vi "Pre Launch Init.vi"(11 "CS++DeviceGUIActor in":refnum<class "CS++DeviceGUIActor.lvclass">) -> (0 "error out":errorcluster, 3 "CS++DeviceGUIActor out":refnum<class "CS++DeviceGUIActor.lvclass">)   [LabVIEW 2013, in "CS++DeviceGUIActor.lvlib" / "CS++DeviceGUIActor.lvclass"]
doc: "(<B>Filename</B>: Actor Framework.lvlib:Actor.lvclass:Pre Launch Init.vi)\n\nDefines behavior that occurs after the Launch Actor method is invoked but before the actor's Actor Core method begins running.\n\nThe Pre Launch Init method is guaranteed to finish before the Launch Actor method returns to its caller and before the actor itself receives any messages. Any references that the Pre Launch Init method obtains are guaranteed to have the same lifetime as the actor itself. Any errors that the Pre Launch Init method returns will abort the launch.\n\nBy default, this method does nothing. A descendant class may override it to define behavior."
uses:
  CS++DeviceGUIActor.lvclass
  CS++GUIActor/CS++GUIActor.lvclass
  CS++BaseActor/CS++BaseActor.lvclass/CS++BaseActor.ctl
  Classes/CS++BaseClasses/Factory/CS++Factory.lvclass
  Classes/CS++ProcessVariables/PVConnection/PVConnection.lvclass
  Classes/CS++ProcessVariables/SVConnection/SVConnection.lvclass
  Classes/CS++ProcessVariables/PVConnection/PVConnection.lvclass/PVConnection.ctl
  Classes/CS++ProcessVariables/ProcessVariable/PV.lvclass/PV.ctl
  CS++DeviceGUIActor.lvclass/CS++DeviceGUIActor.ctl
  Classes/CS++ProcessVariables/ProcessVariable/Read Data.vi
  CS++BaseActor/Read CS++Factory.vi
  Classes/CS++ProcessVariables/ProcessVariable/PV.lvclass
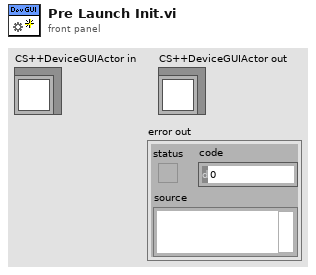
[diagram p1: front panel]
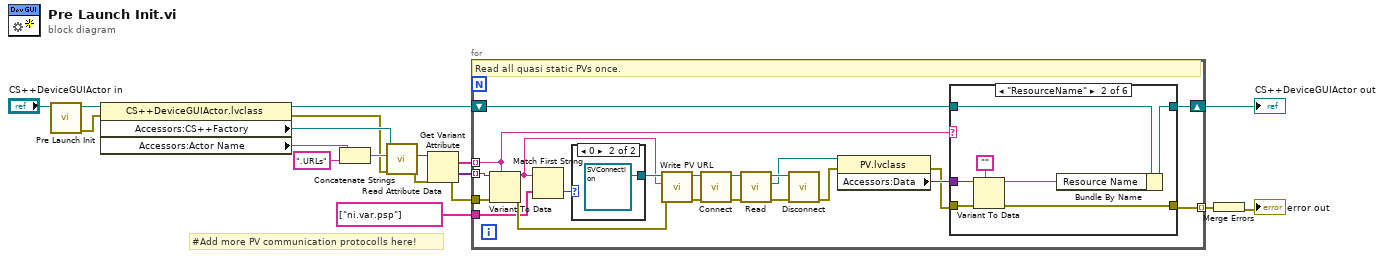
[diagram p0: block diagram]
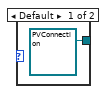
[diagram p2: hidden frame]
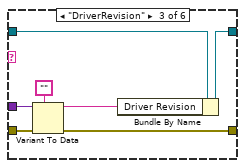
[diagram p4: hidden frame]
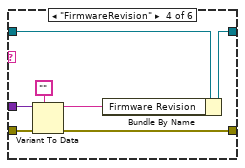
[diagram p5: hidden frame]
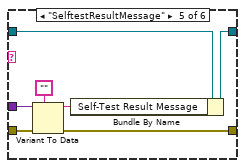
[diagram p6: hidden frame]
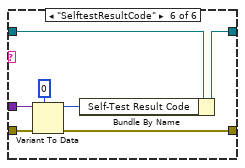
[diagram p7: hidden frame]
diagram:
  # "#Add more PV communication protocolls here!"
  n1 = call-parent "Pre Launch Init.vi"("CS++BaseActor in"="CS++DeviceGUIActor in") -> ("error out"=w4:errorcluster, "CS++BaseActor out"=w5:refnum<class "CS++DeviceGUIActor.lvclass">)  [unwired: 9 in]
  n2 = property class="CS++DeviceGUIActor.lvclass"(reference=w5, error in=w4) -> (reference out=w7:refnum<class "CS++DeviceGUIActor.lvclass">, error out=w14:errorcluster, "Accessors:CS++Factory"=w15:refnum<class "CS++Factory.lvclass">, "Accessors:Actor Name"=w13:string)
  n3 = Concatenate Strings(w13, ".URLs" ("string")) -> (w16:string)
  n4 = call-dynamic "Read Attribute Data.vi"("error in (no error)"=w14, "Object Name"=w16, "CS++Factory in"=w15) -> ("error out"=w11:errorcluster, "Attribute Data"=w12:variant)  [unwired: 6 in, 1 out]
  n5 = Get Variant Attribute(Variant=w12, error in=w11) -> (names=w10:string[], values=w9:variant[], error out=w8:errorcluster)  [unwired: 2 in, 1 out]
  n6 = for {
    tunnel: w10 -> [w24] mode=indexing
    tunnel: w9 -> [w39] mode=indexing
    tunnel: w8 -> [w38]
    shift-right: [w36] -> w3
    shift-left: w7 -> [w37]
    tunnel: [w23] -> w6 mode=indexing
    tunnel: string[] ["ni.var.psp"] ("string array") -> [w19]
    # "Read all quasi static PVs once."
    n7 = Variant To Data(error in=w38, type=w24, Variant=w39) -> (data=w20:string, error out=w33:errorcluster)
    n8 = Match First String(2:w19, 3:w20) -> (0:w21:i32)  [unwired: 1 out]
    n9 = case shown="0" w21 {
      tunnel: [refnum<class "PVConnection.lvclass"> refnum ("CS++ProcessVariables.lvlib:PVConnection.lvclass") refnum<class "SVConnection.lvclass"> refnum ("CS++ProcessVariables.lvlib:SVConnection.lvclass")] -> w22
      frame Default {
      }
      frame 0 {
      }
    }
    n10 = call "Write PV URL.vi"("error in (no error)"=w33, "PV URL"=w20, "PVConnection in"=w22) -> ("error out"=w34:errorcluster, "PVConnection out"=w35:refnum<class "PVConnection.lvclass">)  [unwired: 7 in]
    n11 = call-dynamic "Connect.vi"("error in (no error)"=w34, "PVConnection in"=w35) -> ("error out"=w31:errorcluster, "PVConnection out"=w32:refnum<class "PVConnection.lvclass">)  [unwired: 8 in]
    n12 = call-dynamic "Read.vi"("error in (no error)"=w31, "PVConnection in"=w32) -> ("error out"=w29:errorcluster, "PV"=w28:refnum<class "PV.lvclass">, "PVConnection out"=w30:refnum<class "PVConnection.lvclass">)  [unwired: 7 in]
    n13 = call-dynamic "Disconnect.vi"("error in (no error)"=w29, "PVConnection in"=w30) -> ("error out"=w27:errorcluster)  [unwired: 8 in, 1 out]
    n14 = property class="PV.lvclass"(reference=w28, error in=w27) -> (error out=w25:errorcluster, "Accessors:Data"=w26:variant)  [unwired: 1 out]
    n15 = case shown="\"ResourceName\"" w24 {
      tunnel: w37 -> [w43 w50 w57 w64 w71 w78]
      tunnel: [w43 w49 w56 w63 w70 w77] -> w36
      tunnel: w26 -> [_ w48 w55 w62 w69 w76]
      tunnel: w25 -> [w42 w46 w53 w60 w67 w74]
      tunnel: [w42 w44 w51 w58 w65 w72] -> w23
      frame Default {
      }
      frame "ResourceName" {
        n16 = Variant To Data(error in=w46, type="", Variant=w48) -> (data=w45:string, error out=w44:errorcluster)
        n17 = Bundle By Name(cluster=w50, "Resource Name"=w45) -> (w49:refnum<class "CS++DeviceGUIActor.lvclass">)
      }
      frame "DriverRevision" {
        n18 = Variant To Data(error in=w53, type="", Variant=w55) -> (data=w52:string, error out=w51:errorcluster)
        n19 = Bundle By Name(cluster=w57, "Driver Revision"=w52) -> (w56:refnum<class "CS++DeviceGUIActor.lvclass">)
      }
      frame "FirmwareRevision" {
        n20 = Variant To Data(error in=w60, type="", Variant=w62) -> (data=w59:string, error out=w58:errorcluster)
        n21 = Bundle By Name(cluster=w64, "Firmware Revision"=w59) -> (w63:refnum<class "CS++DeviceGUIActor.lvclass">)
      }
      frame "SelftestResultMessage" {
        n22 = Variant To Data(error in=w67, type="", Variant=w69) -> (data=w66:string, error out=w65:errorcluster)
        n23 = Bundle By Name(cluster=w71, "Self-Test Result Message"=w66) -> (w70:refnum<class "CS++DeviceGUIActor.lvclass">)
      }
      frame "SelftestResultCode" {
        n24 = Variant To Data(error in=w74, type=0, Variant=w76) -> (data=w73:i32, error out=w72:errorcluster)
        n25 = Bundle By Name(cluster=w78, "Self-Test Result Code"=w73) -> (w77:refnum<class "CS++DeviceGUIActor.lvclass">)
      }
    }
  }
  "CS++DeviceGUIActor out" <- w3
  n26 = Merge Errors(w6) -> (→"error out":errorcluster)
